vi "OC2 Setup Test mode.vi"(2 "error in (no error)":errorcluster, 3 "test type values":T1 {"Test Type" items=["Off", "Normal", "Temp Cycle", "Temp Ramp", "Auto Tune"]}, 4 "enable":bool, 5 "VISA resource name":refnum<visa-resource-name>) -> (0 "error out":errorcluster, 1 "dup VISA resource name":refnum<visa-resource-name>)   [LabVIEW 2009]
doc: "TCM set Test mode.vi\n\nVI that sets the test mode information, accepts a cluster that contains the following variables:\nCylce / Time max - \nStart Temp/ Setpoint -\nEnd Temp / end peak test - \nRate 1/calc pid\nRate 2/ run PID\nTime 1/ Undo PID\nTime 2/ Autocal\n\nCOPYRIGHT ELECTRON DYNAMICS LTD"
panel:
  out "write data":string
  # "Set test variables"
  # "V1.02"
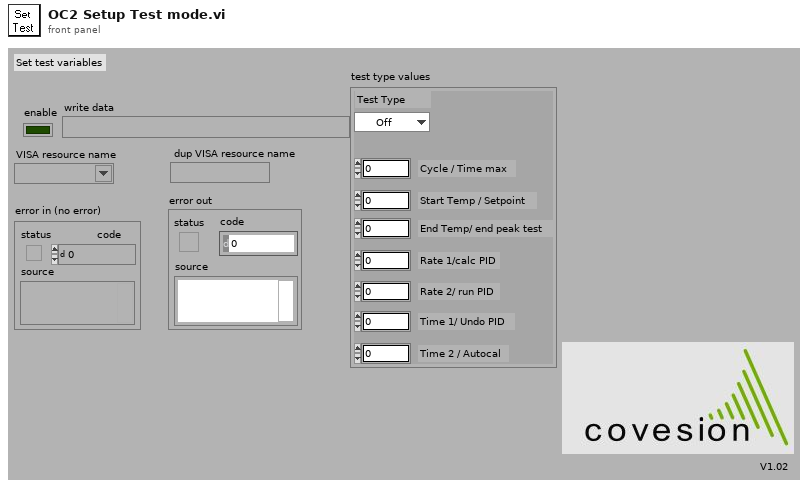
[diagram p1: front panel]
types:
  T1 = cluster{"Test Type ":u16, "Start Temp / Setpoint ":dbl, "End Temp/ end peak test":dbl, "Rate 1/calc PID":dbl, "Rate 2/ run PID":dbl, "Time 1/ Undo PID":dbl, "Time 2 / Autocal":dbl, "Cycle / Time max ":dbl}
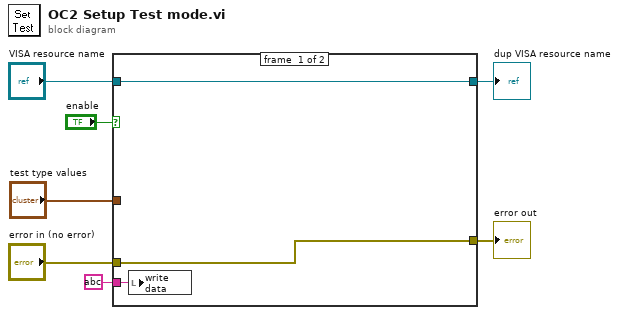
[diagram p0: block diagram]
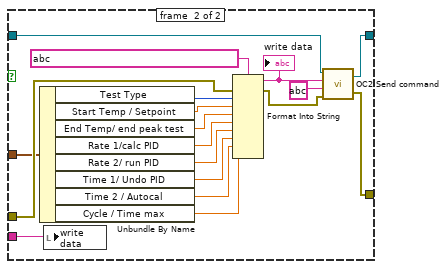
[diagram p2: hidden frame]
diagram:
  n1 = case shown="True" "enable" {
    tunnel: "VISA resource name" -> [w10 w25]
    tunnel: "error in (no error)" -> [w9 w24]
    tunnel: [w9 w22] -> w5
    tunnel: [w10 w21] -> w4
    tunnel: "test type values" -> [_ w20]
    tunnel: string ? -> [w8 w11]
    frame #0 {
      n2 = local write "write data"(w8) -> ()
    }
    frame #1 {
      n3 = Unbundle By Name(w20) -> ("Test Type"=w19:u16, "Start Temp / Setpoint"=w18:dbl, "End Temp/ end peak test"=w17:dbl, "Rate 1/calc PID"=w16:dbl, "Rate 2/ run PID"=w15:dbl, "Time 1/ Undo PID"=w14:dbl, "Time 2 / Autocal"=w13:dbl, "Cycle / Time max"=w12:dbl)
      n4 = local write "write data"(w11) -> ()
      n5 = Format Into String(format string=string ?, error in=w24, w19, w18, w17, w16, w15, w14, w13, w12) -> (resulting string=w26:string, error out=w23:errorcluster)  [unwired: 1 in]
      "write data" <- w26
      n6 = call "OC2 Send command.vi"("VISA resource name"=w25, "Command data"=w26, "Command"=string ?, "error in (no error)"=w23) -> ("dup VISA resource name"=w21:refnum<visa-resource-name>, "error out"=w22:errorcluster)  [unwired: 1 in]
    }
  }
  "dup VISA resource name" <- w4
  "error out" <- w5
